vi "AlliGator Convert Phasor Plot Point to Phasor.vi"(9 "Phasor Plot Reference Points":T3, 11 "Phasor Plot Point":T2) -> (3 "Phasor":T1)   [LabVIEW 2021, in "AlliGator Phasor Plot.lvlib"]
doc: "Converts Phasor Plot image coordinates to actual phasor value."
uses:
  AlliGator Phasor Plot.lvlib
  AlliGator Phasor Plot Reference Points.ctl
  Image/Image Point.ctl
  Phasor/Phasor (g, s).ctl
  Phasor/Phasor.lvlib
  AlliGator Phasor Ratio.lvlib
  Image/Image.lvlib
panel:
  # "see the AlliGator License on the block diagram (Ctrl+E or Window:Show Block Diagram)"
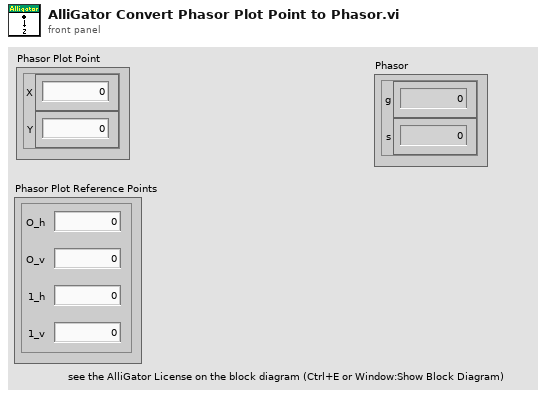
[diagram p1: front panel]
types:
  T1 = typedef "Phasor.lvlib/Phasor (g, s).ctl" = cluster{"g":dbl, "s":dbl}
  T2 = typedef "Image.lvlib/Image Point.ctl" = cluster{"X":i32, "Y":i32}
  T3 = typedef "AlliGator Phasor Ratio.lvlib/AlliGator Phasor Plot Reference Points.ctl" = cluster{"O_h":dbl, "O_v":dbl, "1_h":dbl, "1_v":dbl}
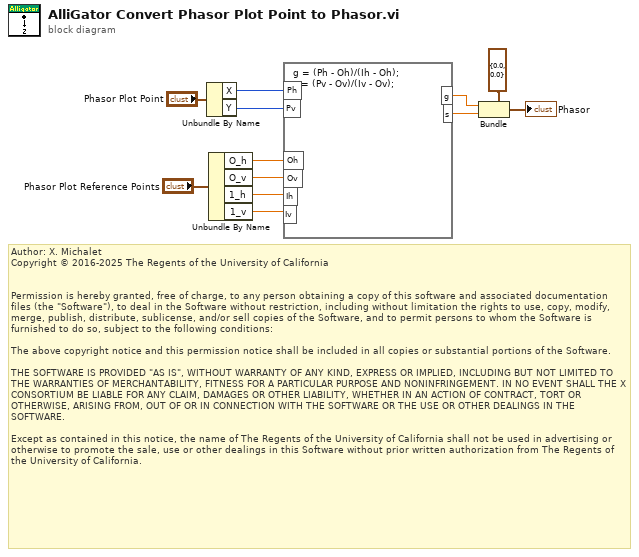
[diagram p0: block diagram]
diagram:
  # "Author: X. Michalet\nCopyright © 2016-2025 The Regents of the University of California\n \n\nPermission is hereby granted, free of charge, to any person obtaining a copy of this software and associated documentation files (the \"Software\"), to deal in the Software without restriction, including without limitation the rights to use, copy, modify, merge, publish, distribute, sublicense, and/or sell copies of the Software, and to permit persons to whom the Software is furnished to do so, subject to the following conditions:\n\nThe above copyright notice and this permission notice shall be included in all copies or substantial portions of the Software.\n\nTHE SOFTWARE IS PROVIDED \"AS IS\", WITHOUT WARRANTY OF ANY KIND, EXPRESS OR IMPLIED, INCLUDING BUT NOT LIMITED TO THE WARRANTIES OF MERCHANTABILITY, FITNESS FOR A PARTICULAR PURPOSE AND NONINFRINGEMENT. IN NO EVENT SHALL THE X CONSORTIUM BE LIABLE FOR ANY CLAIM, DAMAGES OR OTHER LIABILITY, WHETHER IN AN ACTION OF CONTRACT, TORT OR OTHERWISE, ARISING FROM, OUT OF OR IN CONNECTION WITH THE SOFTWARE OR THE USE OR OTHER DEALINGS IN THE SOFTWARE.\n\nExcept as contained in this notice, the name of The Regents of the University of California shall not be used in advertising or otherwise to promote the sale, use or other dealings in this Software without prior written authorization from The Regents of the University of California."
  n1 = Unbundle By Name("Phasor Plot Point") -> ("X"=w10:i32, "Y"=w9:i32)
  n2 = Unbundle By Name("Phasor Plot Reference Points") -> ("O_h"=w8:dbl, "O_v"=w7:dbl, "1_h"=w6:dbl, "1_v"=w5:dbl)
  n3 = formula code="g = (Ph - Oh)/(Ih - Oh);\ns = (Pv - Ov)/(Iv - Ov);"("Ph"=w10, "Pv"=w9, "Oh"=w8, "Ov"=w7, "Ih"=w6, "Iv"=w5) -> ("g"=w3:dbl, "s"=w2:dbl)
  n4 = Bundle(cluster=T1 {"g"=0.0, "s"=0.0} ("Phasor"), "g"=w3, "s"=w2) -> (→"Phasor":T1)
